vi "write_to_db.vi"(0 "reference in":refnum<class "Sig_DA.lvclass">, 11 "error in (no error)":errorcluster) -> (4 "reference out":refnum<class "Sig_DA.lvclass">, 15 "error out":errorcluster)   [LabVIEW 2019, in "Sig_DA.lvclass"]
uses:
  Sig_DA.lvclass
  C:/Users/H4001/Documents/GitHub/H4000/src/Proccess_class/Proccess.lvclass
  Proccess_class/Proccess.lvclass/Proccess.ctl
  Sig_DA.lvclass/Sig_DA.ctl
  Logger_class/Priority.ctl
  Logger_class/EventData.ctl
  Logger_class/EventCode.ctl
  Logger_class/Logger.lvclass
  Proccess_class/Proccess.lvclass
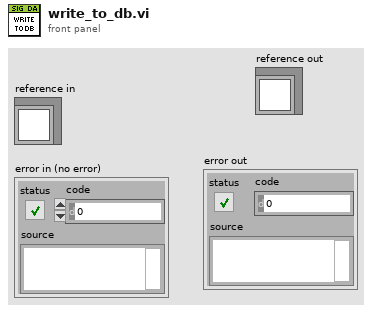
[diagram p1: front panel]
types:
  T1 = typedef "Logger.lvclass/Priority.ctl" = enum16{"Alert", "Critical", "Error", "Warning", "Notice", "Informational", "Debug"}
  T2 = typedef "Logger.lvclass/EventData.ctl" = cluster{"obj_tag":string, "event_tag":string, "code":T3, "Priority":T1, "Value":dbl, "Description":string, "Time Stamp":timestamp}
  T3 = typedef "Logger.lvclass/EventCode.ctl" = enum16{"DI_EU_LO", "DI_EU_HI", "DIO_LO", "DIO_HI", "DI_RAW_LO", "DI_RAW_HI", "DO_LO", "DO_HI", "DA_OK", "DA_ALARM", "AA_HI", "AA_HIHI", "AA_LO", "AA_LOLO", "AA_OK", "CMD", "OUT_OF_RANGE_OK", "OUT_OF_RANGE_LO", "OUT_OF_RANGE_HI", "CONFIG", "DI_LO", "DI_HI"}
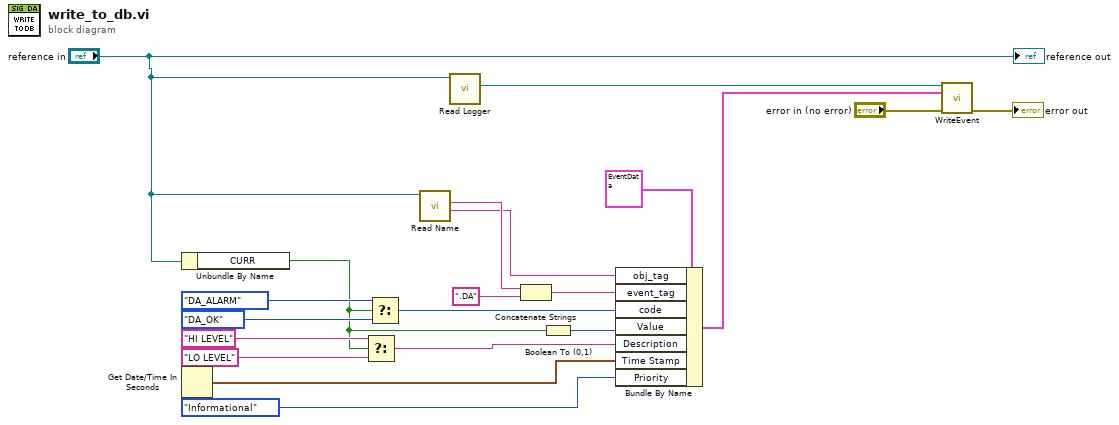
[diagram p0: block diagram]
diagram:
  n1 = Unbundle By Name("reference in") -> ("CURR"=w10:bool)
  n2 = Get Date/Time In Seconds() -> (seconds since 1Jan1904=w7:timestamp)
  n3 = Select(t="HI LEVEL" ("Description"), s=w10, f="LO LEVEL" ("Description")) -> (s? t:f=w8:string)
  n4 = Select(t=EventCode."DA_ALARM" ("code"), s=w10, f=EventCode."DA_OK" ("code")) -> (s? t:f=w13:T3)
  n5 = call "Read Name.vi"("Proccess in"="reference in") -> ("ParentName"=w1:string, "Name"=w4:string)  [unwired: 9 in]
  n6 = call "Read Logger.vi"("Proccess in"="reference in") -> ("Logger"=w3:refnum<class "Logger.lvclass">)  [unwired: 10 in]
  n7 = Concatenate Strings(w4, ".DA" ("string")) -> (w16:string)
  n8 = Boolean To (0,1)(Boolean=w10) -> (0, 1=w12:i16)
  n9 = Bundle By Name(cluster=T2 {"obj_tag"="", "event_tag"="", "code"=enum."DI_RAW_LO", "Priority"=enum."Alert", "Value"=0.0, "Description"="", "Time Stamp"=timestamp(0 s since 1904-01-01)} ("Event"), "obj_tag"=w1, "event_tag"=w16, "code"=w13, "Value"=w12, "Description"=w8, "Time Stamp"=w7, "Priority"=Priority."Informational") -> (w18:T2)
  n10 = call "WriteEvent.vi"("reference in"=w3, "Event"=w18, "error in (no error)"="error in (no error)") -> ("error out"=→"error out":errorcluster)  [unwired: 11 in, 1 out]
  "reference out" <- "reference in"
